vi "robotprofiles.vi"() -> ()   [LabVIEW 2020]
doc: "This global variable contains information that allows similar, but not identical, robots (e.g. an Alpha and a Beta) run identical code bases."
panel:
  out "Robot_Profile":string
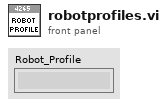
[diagram p1: front panel]
diagram:
